vi "SubLaunch.vi"(8 "error in (no error)":errorcluster, 9 "ID":string, 10 "DeviceObj":refnum<class "Configurable Device.lvclass">, 11 "Controller in":refnum<class "Controller.lvclass">) -> (0 "error out":errorcluster, 3 "Controller out":refnum<class "Controller.lvclass">)   [LabVIEW 2014, in "Controller.lvlib" / "Controller.lvclass"]
doc: "Launches the devices. Devices are launched in parallel. All references to the devices are stored in the Enqueuer MAP and the data map which are both stored in DVRs. This is how we are able to do this in parallel."
uses:
  Controller.lvclass
  Devices/Configurable Device/Configurable Device.lvclass
  SuperActor/Ex Nested.lvclass/Ex Nested.ctl
  Update Controller Data MSG.lvclass
  Messages/Device Init CVT/Device Init CVT MSG.lvclass
  reusable/Session APIs/File Access/Config Data/Config Data.lvclass
  Messages/Update Device Configuration MSG/Update Device Configuration MSG.lvclass
  Devices/Configurable Device/Configurable Device.lvclass/Configurable Device.ctl
  reusable/DAQ Device/Device/Device.lvclass
  reusable/DAQ Device/Device/Generic Data Update Data MSG/Generic Update Data Message.lvclass/Generic Update Data Message.ctl
  reusable/DAQ Device/Device/Device.lvclass/Device.ctl
  reusable/DAQ Device/Device/Write Update Period.vi
  reusable/DAQ Device/Device/Write Configurable Device.vi
  reusable/DAQ Device/Device/Write Update MSG.vi
  SuperActor/Write ID.vi
  reusable/DAQ Device/Device/Write Init CVT MSG.vi
  reusable/DAQ Device/Device/Write Dvc Cfg MSG.vi
  reusable/DAQ Device/Device/Generic Data Update Data MSG/Write ID.vi
  Devices/Configurable Device/Write ID.vi
  SuperActor/Read Config Session.vi
  reusable/Session APIs/File Access/Config Data/Read Array/Read String Array.vi
  <userlib>/_Session Fwk/Session - Root.lvclass
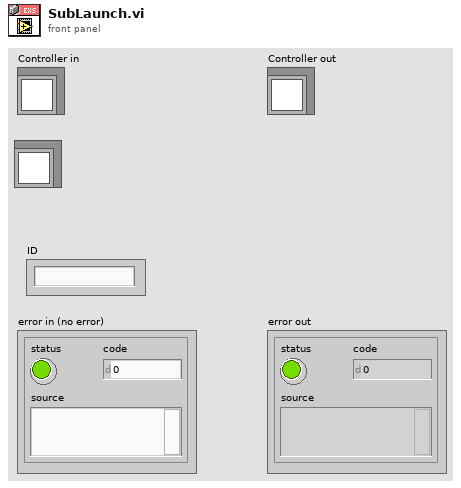
[diagram p1: front panel]
types:
  T1 = typedef "Session - Root.lvclass/Session Handle.ctl" = refnum<data-value>
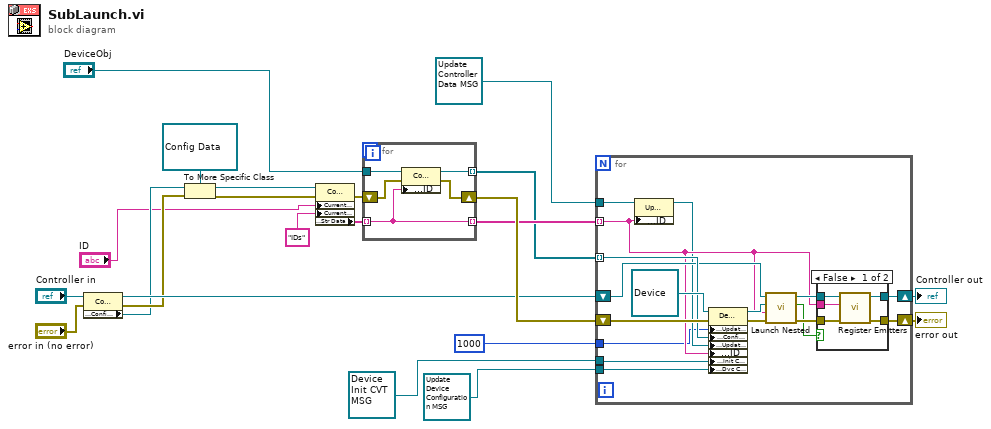
[diagram p0: block diagram]
diagram:
  n1 = property class="Controller"(reference="Controller in", error in="error in (no error)") -> (reference out=w15:refnum<class "Controller.lvclass">, error out=w13:errorcluster, "Accessors:Config Session"=w10:T1)
  n2 = To More Specific Class(target class=refnum<data-value> refnum, reference=w10, error in=w13) -> (specific class reference=w16:refnum<data-value>, error out=w19:errorcluster)
  n3 = property class="Config Data"(reference=w16, error in=w19, "Current Section"="ID", "Current Key"="IDs") -> (error out=w1:errorcluster, "Read Array Data:Str Data"=w2:string[])  [unwired: 1 out]
  n4 = for {
    tunnel: w2 -> [w25] mode=indexing
    tunnel: "DeviceObj" -> [w27]
    tunnel: [w26] -> w17 mode=indexing
    tunnel: [w25] -> w18 mode=indexing
    shift-right: [w24] -> w20
    shift-left: w1 -> [w23]
    n5 = property class="Configurable Device"(reference=w27, error in=w23, "Accessors:ID"=w25) -> (reference out=w26:refnum<class "Configurable Device.lvclass">, error out=w24:errorcluster)
  }
  n6 = for {
    tunnel: w17 -> [w42] mode=indexing
    shift-right: [w35] -> w6
    shift-left: w15 -> [w40]
    tunnel: refnum<class "Update Controller Data MSG.lvclass"> refnum ("Controller.lvlib:Update Data MSG") -> [w41]
    tunnel: w18 -> [w33] mode=indexing
    shift-right: [w34] -> w7
    shift-left: w20 -> [w43]
    tunnel: refnum<class "Device Init CVT MSG.lvclass"> refnum ("Controller.lvlib:Device Init CVT MSG") -> [w31]
    tunnel: refnum<class "Update Device Configuration MSG.lvclass"> refnum ("Controller:Update Device Configuration") -> [w30]
    tunnel: 1000 ("Update Period") -> [w29]
    n7 = property class="Update Data MSG"(reference=w41, "Accessors:ID"=w33) -> (reference out=w32:refnum<class "Update Controller Data MSG.lvclass">)  [unwired: 1 in, 1 out]
    n8 = property class="Device"(reference=refnum<class "Device.lvclass"> refnum ("DAQ Device.lvlib:Device"), error in=w43, "Accessors:Update Period"=w29, "Accessors:Configurable Device"=w42, "Accessors:Update MSG"=w32, "Accessors:ID"=w33, "Accessors:Init CVT MSG"=w31, "Accessors:Dvc Cfg MSG"=w30) -> (reference out=w38:refnum<class "Device.lvclass">, error out=w39:errorcluster)
    n9 = call "Launch Nested.vi"("Error In"=w39, "ID"=w33, "Nested Actor"=w38, "Controller in"=w40) -> ("Error Out"=w36:errorcluster, "Launch Failure?"=w28:bool, "Controller out"=w37:refnum<class "Controller.lvclass">)  [unwired: 5 in]
    n10 = case shown="False" w28 {
      tunnel: w37 -> [w49 w51]
      tunnel: w36 -> [w48 w50]
      tunnel: [w47 w51] -> w35
      tunnel: [w46 w50] -> w34
      tunnel: w33 -> [w45 _]
      frame False {
        n11 = call "Register Emitters.vi"("error in"=w48, "Emitter"=w45, "Controller in"=w49) -> ("error out"=w46:errorcluster, "Controller out"=w47:refnum<class "Controller.lvclass">)  [unwired: 7 in]
      }
      frame True {
      }
    }
  }
  "error out" <- w7
  "Controller out" <- w6
